vi "Fetch STR data.vi"(4 "error in (no error)":errorcluster, 6 "Buffer Size":i32, 7 "Statement Refnum":T1) -> (0 "error out":errorcluster, 1 "String Length":i32, 2 "Data":string, 3 "Statement Refnum":T1)   [LabVIEW 2011]
doc: "Lit la donnée de type string"
uses:
  SQL Controls/Statement Refnum.ctl
  Odbc32.dll
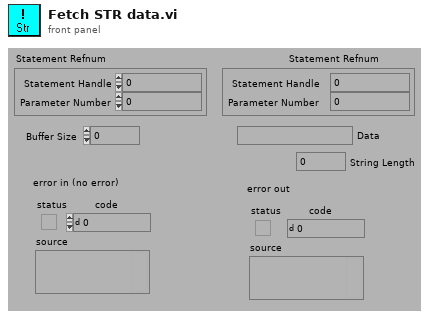
[diagram p1: front panel]
types:
  T1 = typedef "Statement Refnum.ctl" = cluster{"Statement Handle":i32, "Parameter Number":u16}
  T2 = enum16{"NOPE", "SQL_HANDLE_ENV", "SQL_HANDLE_DBC", "SQL_HANDLE_STMT", "SQL_HANDLE_DESC"}
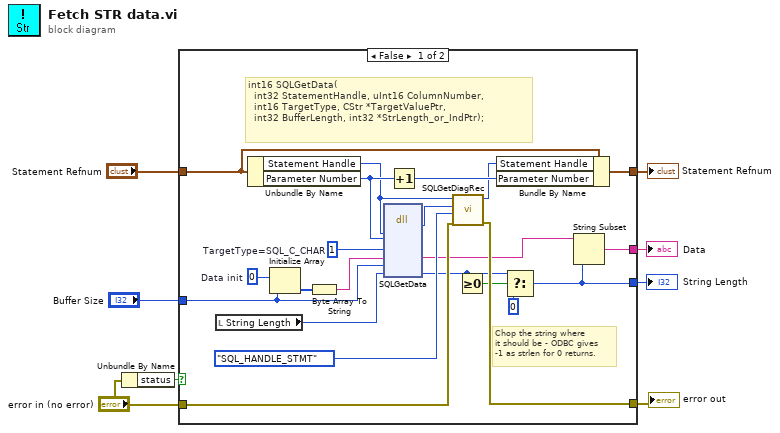
[diagram p0: block diagram]
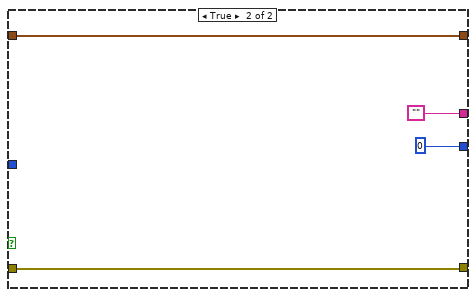
[diagram p2: hidden frame]
diagram:
  n1 = Unbundle By Name("error in (no error)") -> ("status"=w1:bool)
  n2 = case shown="False" w1 {
    tunnel: [w16 ""] -> w8
    tunnel: "Statement Refnum" -> [w30 w31]
    tunnel: [w29 w31] -> w6
    tunnel: "Buffer Size" -> [w15 _]
    tunnel: [w11 0] -> w4
    tunnel: "error in (no error)" -> [w19 w32]
    tunnel: [w18 w32] -> w3
    frame False {
      w23 = i16 1  # TargetType=SQL_C_CHAR
      w26 = u8 0  # Data init
      # "Chop the string where\nit should be - ODBC gives\n-1 as strlen for 0 returns."
      # "int16 SQLGetData(\n  int32 StatementHandle, uInt16 ColumnNumber, \n  int16 TargetType, CStr *TargetValuePtr,\n  int32 BufferLength, int32 *StrLength_or_IndPtr);"
      n3 = local read "String Length"() -> (w9:i32)
      n4 = Unbundle By Name(w30) -> ("Statement Handle"=w21:i32, "Parameter Number"=w28:u16)
      n5 = Initialize Array(w26, w15) -> (w25:u8[])
      n6 = Byte Array To String(unsigned byte array=w25) -> (string=w24:string)
      n7 = dll-call lib="Odbc32.dll" fn="SQLGetData"("StatementHandle"=w21, "ColumnNumber"=w28, "TargetType"=w23, "TargetValuePtr"=w24, "BufferLength"=w15, "StrLength_or_IndPtr"=w9) -> (w22:i16, "TargetValuePtr"=w10:string, "StrLength_or_IndPtr"=w13:i32)  [unwired: 7 in, 2 out]
      n8 = Increment(x=w28) -> (x+1=w27:u16)
      n9 = call "SQLGetDiagRec.vi"("error in (no error)"=w19, "HandleType"=T2."SQL_HANDLE_STMT", "Status (SQL_SUCCESS=0)"=w22, "Input Handle"=w21) -> ("error out"=w18:errorcluster, "Output Handle"=w20:i32)  [unwired: 2 out]
      n10 = Greater Or Equal To 0?(x=w13) -> (x >= 0?=w14:bool)
      n11 = Bundle By Name(cluster=w30, "Statement Handle"=w20, "Parameter Number"=w27) -> (w29:T1)
      n12 = Select(t=w13, s=w14, f=0) -> (s? t:f=w11:i32)
      n13 = String Subset(string=w10, length (rest)=w11) -> (substring=w16:string)  [unwired: 1 out]
    }
    frame True {
    }
  }
  "Statement Refnum" <- w6
  "Data" <- w8
  "String Length" <- w4
  "error out" <- w3
